vi "LI-U8 convert U32 to U8 array number.vi"(4 "U32":u32) -> (1 "Large number -U8":T1)   [LabVIEW 2012]
doc: "Converts a U32 to large integer in U8 array format ."
uses:
  User Access Type defs/Large number - U8 array.ctl
panel:
  # "<<LSD"
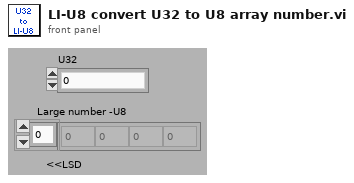
[diagram p1: front panel]
types:
  T1 = typedef "Large number - U8 array.ctl" = u8[]
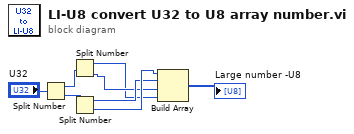
[diagram p0: block diagram]
diagram:
  n1 = Split Number(x="U32") -> (hi(x)=w7:u16, lo(x)=w6:u16)
  n2 = Split Number(x=w7) -> (hi(x)=w2:u8, lo(x)=w3:u8)
  n3 = Split Number(x=w6) -> (hi(x)=w4:u8, lo(x)=w5:u8)
  n4 = Build Array(w5, w4, w3, w2) -> (→"Large number -U8":u8[])
